vi "Set Event Measurement Properties.vi"(8 "error in (no error)":errorcluster, 10 "measurement":T1={"Name"="", "Bitfile name"="", "Window"="", "Polarity"=enum."Active high"}, 11 "Item Ref in":T3 format="%.0x") -> (0 "error out":errorcluster, 2 "failed":bool, 3 "Item Ref out":T3 format="%.0x")   [LabVIEW 2020, in "Engine Simulation Toolkit System Explorer.lvlib"]
uses:
  Engine Simulation Toolkit System Explorer.lvlib
  <vilib>/NI VeriStand/Custom Device API/Custom Device Item Ref.ctl
  Event Timing Measurement.ctl
  Polarity.ctl
  Shared/Properties.vi
  <vilib>/NI VeriStand/Custom Device Tools/Custom Device Utility Library/NI VeriStand - Search for Item by Property.vi
  <vilib>/NI VeriStand/Custom Device API/Set Item Property (String).vi
  <vilib>/NI VeriStand/Custom Device API/Set Item Property (U16).vi
  <vilib>/NI VeriStand/Custom Device API/Custom Device API.lvlib
  Shared/Engine Simulation Toolkit Shared.lvlib
  <vilib>/NI VeriStand/Custom Device Tools/Custom Device Utility Library/Custom Device Utility Library.lvlib
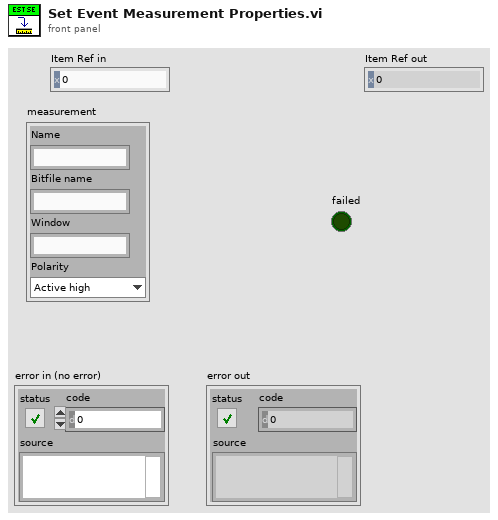
[diagram p1: front panel]
types:
  T1 = typedef "Engine Simulation Toolkit System Explorer.lvlib/Event Timing Measurement.ctl" = cluster{"Name":string, "Bitfile name":string, "Window":string, "Polarity":T2}
  T2 = typedef "Engine Simulation Toolkit System Explorer.lvlib/Polarity.ctl" = enum16{"Active low", "Active high"}
  T3 = typedef "Custom Device API.lvlib/Custom Device Item Ref.ctl" = u64
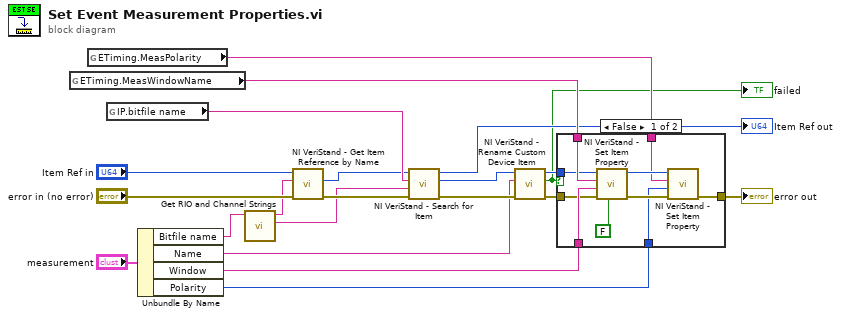
[diagram p0: block diagram]
diagram:
  n1 = global read "Properties.vi" "ETiming.MeasWindowName"() -> (w20:string)
  n2 = global read "Properties.vi" "ETiming.MeasPolarity"() -> (w14:string)
  n3 = global read "Properties.vi" "IP.bitfile name"() -> (w5:string)
  n4 = Unbundle By Name("measurement") -> ("Bitfile name"=w2:string, "Name"=w10:string, "Window"=w16:string, "Polarity"=w15:T2)
  n5 = call "Get RIO and Channel Strings.vi"("rio/channel"=w2) -> ("channel"=w3:string, "rio"=w4:string)  [unwired: 9 in]
  n6 = call <vilib>:"NI VeriStand - Get Item Reference by Name.vi"("error in (no error)"="error in (no error)", "Item Name"=w4, "Parent Ref in"="Item Ref in") -> ("error out"=w6:errorcluster, "Item Ref"=w1:T3)  [unwired: 5 in, 2 out]
  n7 = call-poly <vilib>:"NI VeriStand - Search for Item.vi"("error in"=w6, "Property Value"=w3, "Property Name"=w5, "Section Ref in"=w1) -> ("error out"=w18:errorcluster, "Item Ref"=w12:T3, "Section Ref out"=→"Item Ref out":T3)  [unwired: 4 in, 1 out]
  n8 = call <vilib>:"NI VeriStand - Rename Custom Device Item.vi"("error in (no error)"=w18, "New Name"=w10, "Item Ref in"=w12) -> ("error out"=w13:errorcluster, "Request invalid?"=w9:bool, "Item Ref out"=w11:T3)  [unwired: 6 in]
  "failed" <- w9
  n9 = case shown="False" w9 {
    tunnel: [w30 w32] -> w21
    tunnel: w20 -> [w28 _]
    tunnel: w16 -> [w27 _]
    tunnel: w15 -> [w26 _]
    tunnel: w14 -> [w25 _]
    tunnel: w13 -> [w24 w32]
    tunnel: w11 -> [w23 _]
    frame False {
      n10 = call-poly <vilib>:"NI VeriStand - Set Item Property.vi"("Binary String (T)"=FALSE, "error in (no error)"=w24, "Value"=w27, "Property Name"=w28, "Item Ref in"=w23) -> ("error out"=w31:errorcluster, "Item Ref out"=w29:T3)  [unwired: 4 in, 1 out]
      n11 = call-poly <vilib>:"NI VeriStand - Set Item Property.vi"("error in (no error)"=w31, "Value"=w26, "Property Name"=w25, "Item Ref in"=w29) -> ("error out"=w30:errorcluster)  [unwired: 5 in, 2 out]
    }
    frame True {
    }
  }
  "error out" <- w21
